vi "XY_coordinate.vi"(7 "stc_TimeInit":T4) -> (0 "str_ElapsedTime":string, 1 "str_2ndLineTime":string, 2 "str_1stLineTime":string, 3 "XY_Coordinate":picture, 4 "str_RunningTime":string, 8 "ms16EachXYHigh":i16, 9 "mu08ObjectNum":u8, 10 "mu08XOffset":u8, 11 "stc_NumOffset":cluster{"XOffset":u8, "YOffset":u8})   [LabVIEW 2011]
uses:
  <vilib>/picture/picture.llb/imagedata.ctl
panel:
  out "大小":i32
  out "image data":T1 caption="图像数据"
  out "PicJpgPath":path
  out "mbfUpdate":bool
  in  "ClearRedBlueLine":bool
  out "stc_absLine":cluster{"absTop":u8, "absBotton":u16}
  out "stc_BlueLineBK":T2
  out "stc_RedLineBK":T2
  out "stc_XYOriginOffset":T3
  out "stc_BlueLine":T2
  out "stc_RedLine":T2
  out "strInputInit":string
  out "Pic_Right":u32
  out "Pic_Left":i32
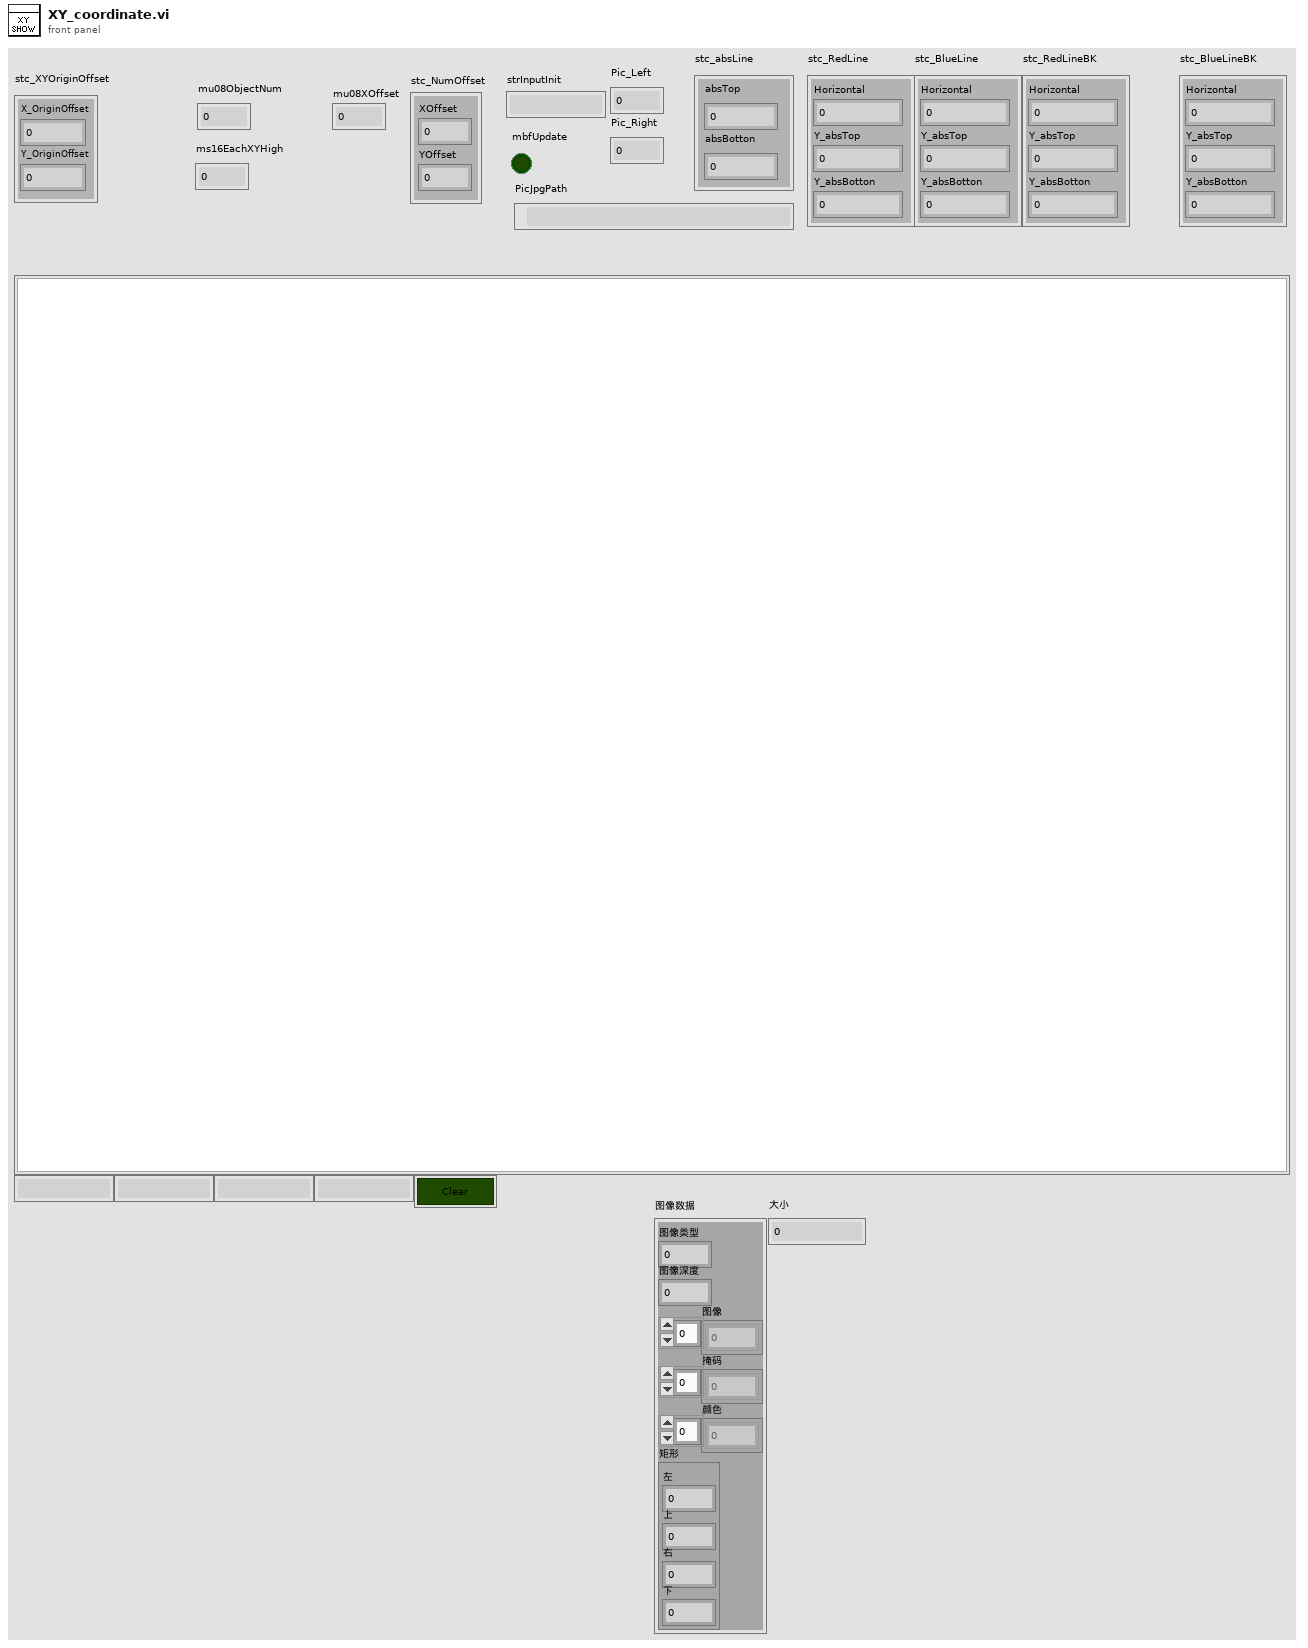
[diagram p1: front panel]
types:
  T1 = typedef "imagedata.ctl" = cluster{"image type":i32, "image depth":i32, "image":u8[], "mask":u8[], "colors":u32[], "Rectangle":cluster{"left":i16, "top":i16, "right":i16, "bottom":i16}}
  T2 = cluster{"Horizontal":u32, "Y_absTop":u8, "Y_absBotton":u16}
  T3 = cluster{"X_OriginOffset":u8, "Y_OriginOffset":dbl}
  T4 = cluster{"str_1stLineTime":string, "str_2ndLineTime":string, "str_ElapsedTime":string, "str_RunningTime":string}
  T5 = cluster{"Width":u16, "Style":enum32{"Solid", "Dash", "Dot", "DashDot", "DashDotDot"}}
  T6 = typedef "LVBoundsTypeDef.ctl" = cluster{"Width":u32, "Height":u32}
  T7 = typedef "LVPoint32TypeDef.ctl" = cluster{"Horizontal":i32, "Vertical":i32}
  T8 = cluster{"Shift":bool, "Ctrl":bool, "Alt":bool, "Cmd":bool, "Opt":bool}
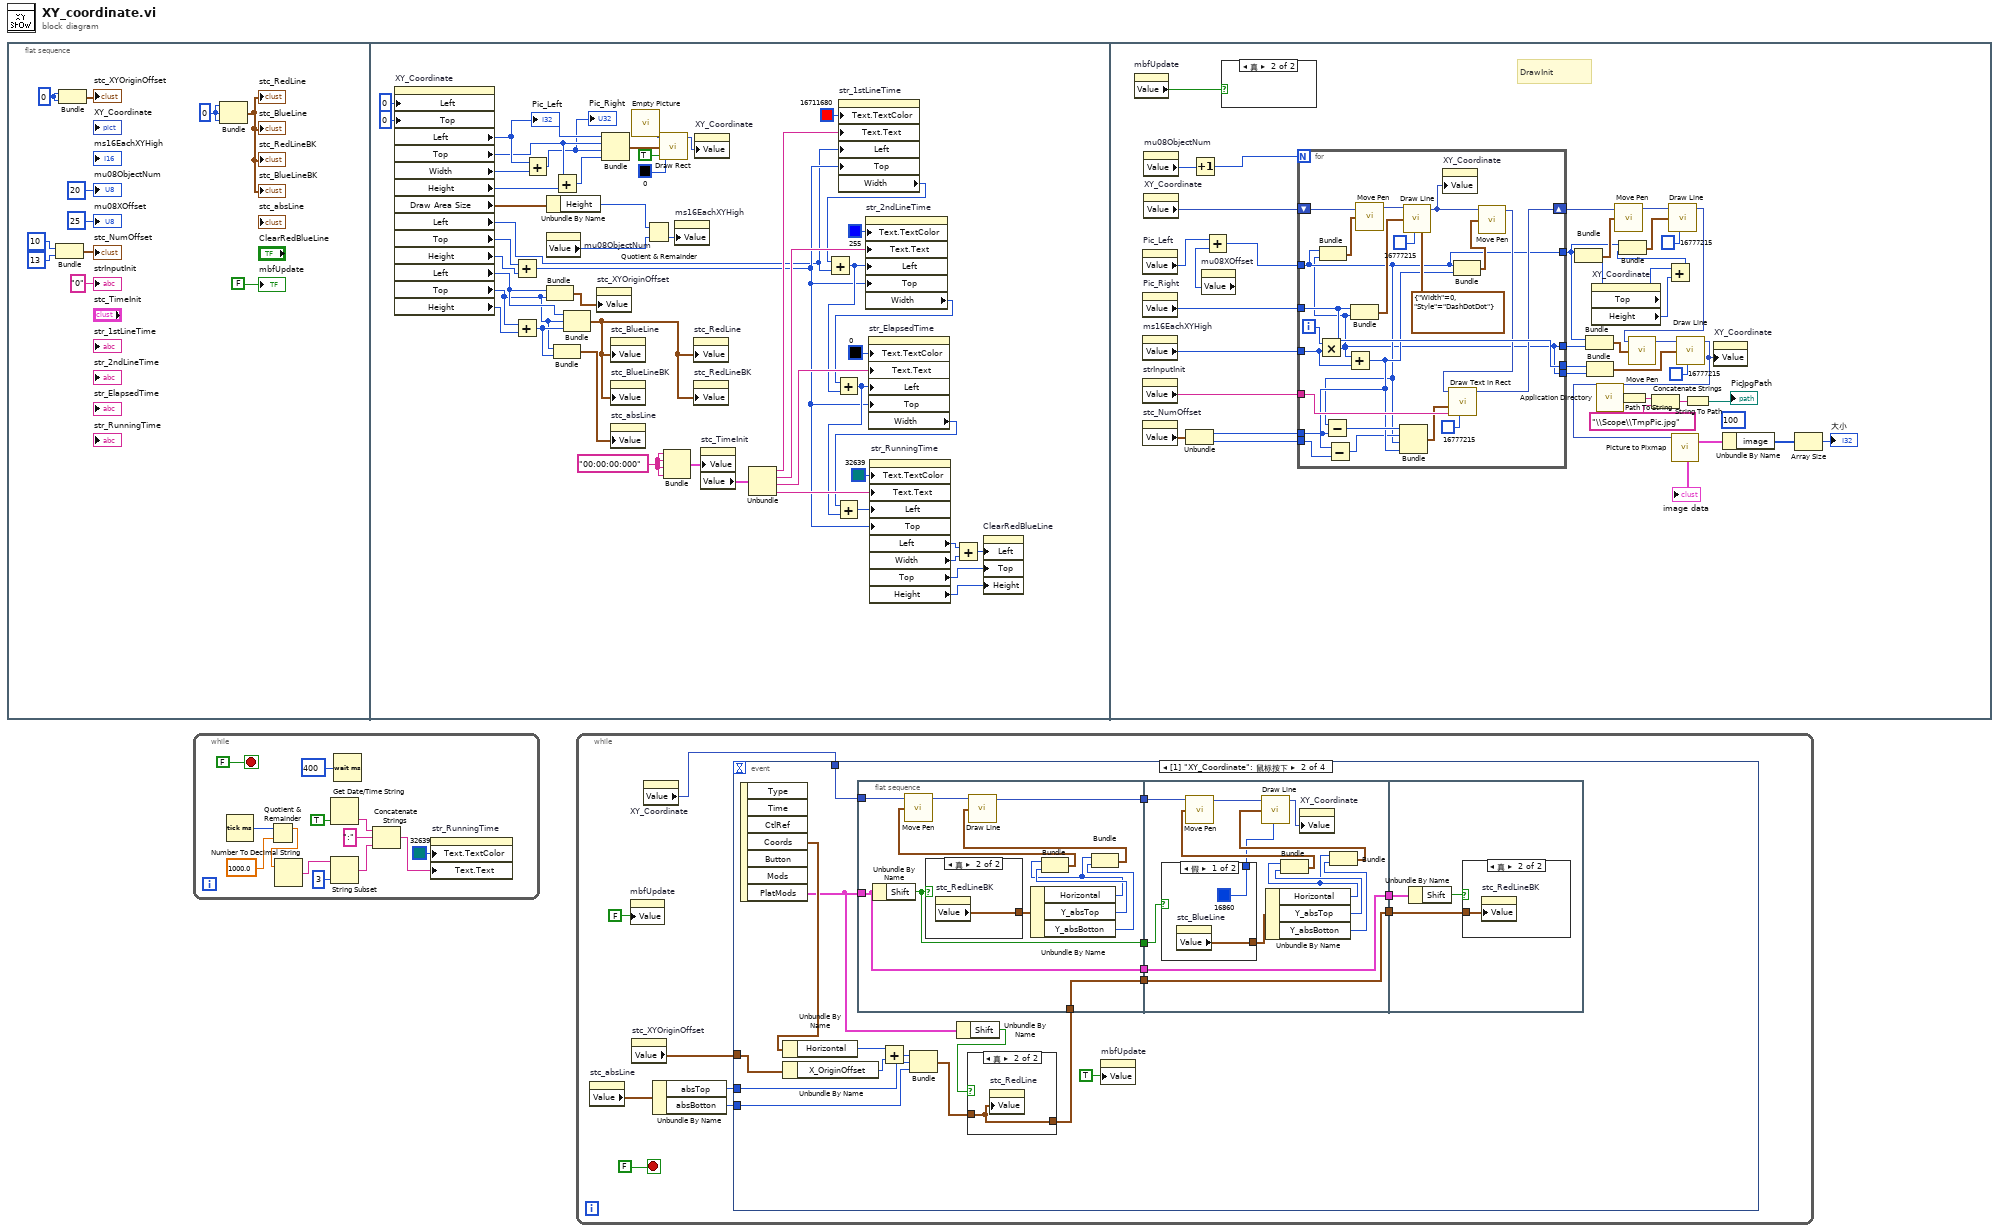
[diagram p0: block diagram]
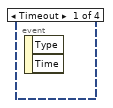
[diagram p2: hidden frame]
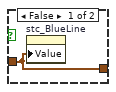
[diagram p3: hidden frame]
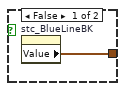
[diagram p4: hidden frame]
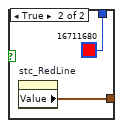
[diagram p5: hidden frame]
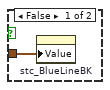
[diagram p6: hidden frame]
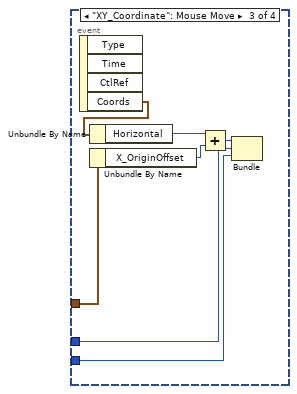
[diagram p7: hidden frame]
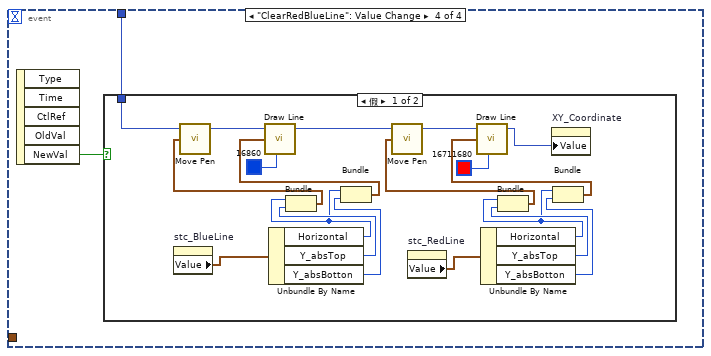
[diagram p8: hidden frame]
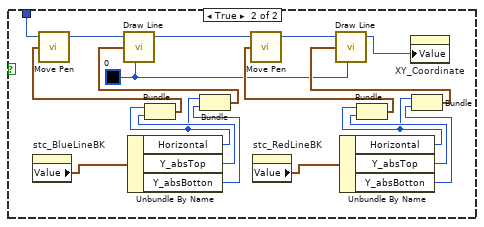
[diagram p9: hidden frame]
diagram:
  n1 = flat-sequence {
    frame #0 {
      w5 = 0
      w3 = 0
      n2 = Bundle(10, 13) -> (→"stc_NumOffset":cluster{i32, i32})  [unwired: 1 in]
      n3 = Bundle(w5, w5) -> (→"stc_XYOriginOffset":cluster{i32, i32})  [unwired: 1 in]
      n4 = Bundle(w3, w3, w3) -> (→"stc_RedLine" →"stc_BlueLine" →"stc_RedLineBK" →"stc_BlueLineBK":cluster{i32, i32, i32})  [unwired: 1 in]
      "mu08ObjectNum" <- u8 20 ("mu08ObjectNum")
      "mu08XOffset" <- u8 25 ("mu08XBuf")
      "strInputInit" <- "0" ("strInputInit")
      "mbfUpdate" <- FALSE
    }
    frame #1 {
      w43 = "00:00:00:000"
      n5 = property on="XY_Coordinate" class="Pict"("Left"=0 ("位置:居左"), "Top"=0 ("位置:置顶")) -> ("Left"=w58:i32, "Top"=w55:i32, "Width"=w57:u32, "Height"=w56:u32, "Draw Area Size"=w49:T6, "Left"=w19:i32, "Top"=w44:i32, "Height"=w18:u32, "Left"=w24:i32, "Top"=w20:i32, "Height"=w17:u32)  [unwired: 2 in, 2 out]
      "Pic_Left" <- w58
      n6 = Add(x=w44, y=w18) -> (x+y=w26:u32)
      n7 = Add(x=w20, y=w17) -> (x+y=w22:u32)
      n8 = Add(x=w58, y=w57) -> (x+y=w45:u32)
      "Pic_Right" <- w45
      n9 = Unbundle By Name(w49) -> ("Height"=w48:u32)
      n10 = property on="mu08ObjectNum" class="DigNum (严格)"() -> ("Value"=w47:u8)  [unwired: 2 in, 2 out]
      n11 = Bundle("Left"=w24, "Top"=w20) -> (w25:cluster{"Left":i32, "Top":i32})  [unwired: 1 in]
      n12 = Add(x=w55, y=w56) -> (x+y=w54:u32)
      n13 = Bundle("Top"=w20, w22) -> (w21:cluster{"Top":i32, u32})  [unwired: 1 in]
      n14 = Bundle("Left"=w24, "Top"=w20, w22) -> (w23:cluster{"Left":i32, "Top":i32, u32})  [unwired: 1 in]
      n15 = property on="stc_XYOriginOffset" class="Clust (严格)"("Value"=w25) -> ()  [unwired: 2 in, 2 out]
      n16 = Bundle("Left"=w58, "Top"=w55, w45, w54) -> (w53:cluster{"Left":i32, "Top":i32, u32, u32})  [unwired: 1 in]
      n17 = property on="stc_BlueLine" class="Clust (严格)"("Value"=w23) -> ()  [unwired: 2 in, 2 out]
      n18 = property on="stc_BlueLineBK" class="Clust (严格)"("Value"=w23) -> ()  [unwired: 2 in, 2 out]
      n19 = property on="stc_absLine" class="Clust (严格)"("Value"=w21) -> ()  [unwired: 2 in, 2 out]
      n20 = call "Empty Picture"() -> ("empty picture"=w59:picture)
      n21 = Quotient & Remainder(x=w48, y=w47) -> (floor(x/y)=w46:u32)  [unwired: 1 out]
      n22 = call <vilib>:"Draw Rect.vi"("picture"=w59, "rect"=w53, "fill?(F)"=TRUE, "color(black)"=u32 0) -> ("new picture"=w50:picture)  [unwired: 5 in]
      n23 = Bundle(w43, w43, w43, w43) -> (w42:cluster{string, string, string, string})  [unwired: 1 in]
      n24 = property on="ms16EachXYHigh" class="DigNum (严格)"("Value"=w46) -> ()  [unwired: 2 in, 2 out]
      n25 = property on="stc_RedLine" class="Clust (严格)"("Value"=w23) -> ()  [unwired: 2 in, 2 out]
      n26 = property on="stc_RedLineBK" class="Clust (严格)"("Value"=w23) -> ()  [unwired: 2 in, 2 out]
      n27 = property on="XY_Coordinate" class="Pict"("Value"=w50) -> ()  [unwired: 2 in, 2 out]
      n28 = property on="stc_TimeInit" class="Clust (严格)"("Value"=w42) -> ("Value"=w41:T4)  [unwired: 2 in, 2 out]
      n29 = Unbundle(w41) -> ("str_1stLineTime"=w36:string, "str_2ndLineTime"=w35:string, "str_ElapsedTime"=w34:string, "str_RunningTime"=w33:string)
      n30 = property on="str_1stLineTime" class="Str"("Text.TextColor"=u32 16711680, "Text.Text"=w36, "Left"=w19, "Top"=w26) -> ("Width"=w32:u32)  [unwired: 2 in, 2 out]
      n31 = Add(x=w32, y=w19) -> (x+y=w30:u32)
      n32 = property on="str_2ndLineTime" class="Str"("Text.TextColor"=u32 255, "Text.Text"=w35, "Left"=w30, "Top"=w26) -> ("Width"=w31:u32)  [unwired: 2 in, 2 out]
      n33 = Add(x=w31, y=w30) -> (x+y=w27:u32)
      n34 = property on="str_ElapsedTime" class="Str"("Text.TextColor"=u32 0, "Text.Text"=w34, "Left"=w27, "Top"=w26) -> ("Width"=w28:u32)  [unwired: 2 in, 2 out]
      n35 = Add(x=w28, y=w27) -> (x+y=w29:u32)
      n36 = property on="str_RunningTime" class="Str"("Text.TextColor"=u32 32639, "Text.Text"=w33, "Left"=w29, "Top"=w26) -> ("Left"=w15:i32, "Width"=w16:u32, "Top"=w13:i32, "Height"=w12:u32)  [unwired: 2 in, 2 out]
      n37 = Add(x=w15, y=w16) -> (x+y=w14:u32)
      n38 = property on="ClearRedBlueLine" class="Bool"("Left"=w14, "Top"=w13, "Height"=w12) -> ()  [unwired: 2 in, 2 out]
    }
    frame #2 {
      (unwired) 100 ("quality (80)")
      # "DrawInit"
      n39 = property on="mbfUpdate" class="Bool (严格)"() -> ("Value"=w100:bool)  [unwired: 2 in, 2 out]
      n40 = property on="Pic_Left" class="DigNum (严格)"() -> ("Value"=w96:i32)  [unwired: 2 in, 2 out]
      n41 = property on="Pic_Right" class="DigNum (严格)"() -> ("Value"=w99:u32)  [unwired: 2 in, 2 out]
      n42 = property on="ms16EachXYHigh" class="DigNum (严格)"() -> ("Value"=w98:i16)  [unwired: 2 in, 2 out]
      n43 = property on="strInputInit" class="Str"() -> ("Value"=w78:string)  [unwired: 2 in, 2 out]
      n44 = property on="stc_NumOffset" class="Clust (严格)"() -> ("Value"=w75:cluster{"XOffset":u8, "YOffset":u8})  [unwired: 2 in, 2 out]
      n45 = property on="mu08ObjectNum" class="DigNum (严格)"() -> ("Value"=w77:u8)  [unwired: 2 in, 2 out]
      n46 = property on="XY_Coordinate" class="Pict"() -> ("Value"=w71:picture)  [unwired: 2 in, 2 out]
      n47 = Unbundle(w75) -> ("XOffset"=w74:u8, "YOffset"=w73:u8)
      n48 = Increment(x=w77) -> (x+1=w76:u8)
      n49 = property on="mu08XOffset" class="DigNum (严格)"() -> ("Value"=w97:u8)  [unwired: 2 in, 2 out]
      n50 = Add(x=w96, y=w97) -> (x+y=w95:i32)
      n51 = case shown="真" w100 {
        frame False {
        }
        frame True {
        }
      }
      n52 = for {
        N: w76 -> [_]
        shift-right: [w116] -> w93
        shift-left: w71 -> [w103]
        tunnel: w95 -> [w105]
        tunnel: w99 -> [w117]
        tunnel: w98 -> [w119]
        tunnel: [w105] -> w85
        tunnel: [w104] -> w83
        tunnel: [w117] -> w82
        tunnel: [w104] -> w81
        tunnel: w78 -> [w114]
        tunnel: [w112] -> _
        tunnel: w74 -> [w112]
        tunnel: w73 -> [w110]
        i -> [w123]
        n53 = Multiply(x=w123, y=w119) -> (x*y=w104:i32)
        n54 = Bundle(w105, w104) -> (w101:cluster{i32, i32})  [unwired: 1 in]
        n55 = Subtract(x=w105, y=w112) -> (x-y=w111:i32)
        n56 = Add(x=w104, y=w119) -> (x+y=w109:i32)
        n57 = Subtract(x=w109, y=w110) -> (x-y=w108:i32)
        n58 = Bundle("Value"=w117, w104) -> (w118:cluster{"Value":u32, i32})  [unwired: 1 in]
        n59 = call <vilib>:"Move Pen.vi"("new position"=w101, "picture"=w103) -> ("new picture"=w102:picture)  [unwired: 3 in]
        n60 = Bundle(w111, w108, w105, w109) -> (w107:cluster{i32, i32, i32, i32})  [unwired: 1 in]
        n61 = call <vilib>:"Draw Line.vi"("picture"=w102, "end point"=w118, "color(black)"=u32 16777215, "pen"=T5 {"Width"=0, "Style"=enum."DashDotDot"}) -> ("new picture"=w121:picture)  [unwired: 5 in]
        n62 = property on="XY_Coordinate" class="Pict"("Value"=w121) -> ()  [unwired: 2 in, 2 out]
        n63 = Bundle(w105, w109) -> (w106:cluster{i32, i32})  [unwired: 1 in]
        n64 = call <vilib>:"Move Pen.vi"("new position"=w106, "picture"=w121) -> ("new picture"=w113:picture)  [unwired: 3 in]
        n65 = call <vilib>:"Draw Text in Rect.vi"("text color(black)"=u32 16777215 ("color(black)"), "text"=w114, "rect"=w107, "picture"=w113) -> ("new picture"=w116:picture)  [unwired: 7 in]
      }
      n66 = Bundle(w85, w83) -> (w80:cluster{i32, i32})  [unwired: 1 in]
      n67 = Bundle("Value"=w82, w81) -> (w79:cluster{"Value":u32, i32})  [unwired: 1 in]
      n68 = property on="XY_Coordinate" class="Pict"() -> ("Top"=w90:i32, "Height"=w87:u32)  [unwired: 2 in, 2 out]
      n69 = Bundle(w85, "Top"=w90) -> (w91:cluster{i32, "Top":i32})  [unwired: 1 in]
      n70 = call <vilib>:"Application Directory.vi"() -> ("Application Directory"=w69:path)
      n71 = call <vilib>:"Move Pen.vi"("new position"=w91, "picture"=w93) -> ("new picture"=w92:picture)  [unwired: 3 in]
      n72 = Path To String(path=w69) -> (string=w68:string)
      n73 = Concatenate Strings(w68, "\\Scope\\TmpPic.jpg") -> (w66:string)
      n74 = Add(x=w90, y=w87) -> (x+y=w88:u32)
      n75 = Bundle(w85, w88) -> (w89:cluster{i32, u32})  [unwired: 1 in]
      n76 = call <vilib>:"Draw Line.vi"("picture"=w92, "end point"=w89, "color(black)"=u32 16777215) -> ("new picture"=w72:picture)  [unwired: 6 in]
      n77 = call <vilib>:"Move Pen.vi"("new position"=w80, "picture"=w72) -> ("new picture"=w86:picture)  [unwired: 3 in]
      n78 = call <vilib>:"Draw Line.vi"("picture"=w86, "end point"=w79, "color(black)"=u32 16777215) -> ("new picture"=w70:picture)  [unwired: 6 in]
      n79 = call <vilib>:"Picture to Pixmap.vi"("picture"=w70) -> ("image data"=w64:T1)  [unwired: 9 in, 1 out]
      "image data" <- w64
      n80 = String To Path(string=w66) -> (path=→"PicJpgPath":path)
      n81 = property on="XY_Coordinate" class="Pict"("Value"=w70) -> ()  [unwired: 2 in, 2 out]
      n82 = Unbundle By Name(w64) -> ("image"=w63:u8[])
      n83 = Array Size(array=w63) -> (size(s)=→"大小":i32)
    }
  }
  n84 = while {
    stop <- FALSE stop-if-true
    n85 = Tick Count (ms)() -> (millisecond timer value=w125:u32)
    n86 = Quotient & Remainder(x=w125, y=1000.0) -> (x-y*floor(x/y)=w124:dbl)  [unwired: 1 out]
    n87 = Number To Decimal String(number=w124) -> (decimal integer string=w135:string)  [unwired: 1 in]
    n88 = Get Date/Time String(want seconds? (F)=TRUE ("需要秒？(F)")) -> (time string=w132:string)  [unwired: 2 in, 1 out]
    n89 = String Subset(string=w135, length (rest)=3 ("长度（剩余）")) -> (substring=w127:string)  [unwired: 1 in]
    n90 = Wait (ms)(milliseconds to wait=u32 400 ("等待时间（毫秒）")) -> ()  [unwired: 1 out]
    n91 = Concatenate Strings(w132, ":" ("字符串"), w127) -> (w130:string)
    n92 = property on="str_RunningTime" class="Str"("Text.TextColor"=u32 32639, "Text.Text"=w130) -> ()  [unwired: 2 in, 2 out]
  }
  n93 = while {
    stop <- FALSE stop-if-true
    n94 = property on="stc_absLine" class="Clust (严格)"() -> ("Value"=w141:cluster{"absTop":u8, "absBotton":u16})  [unwired: 2 in, 2 out]
    n95 = property on="mbfUpdate" class="Bool (严格)"("Value"=FALSE ("mbfUpdate")) -> ()  [unwired: 2 in, 2 out]
    n96 = property on="stc_XYOriginOffset" class="Clust (严格)"() -> ("Value"=w142:T3)  [unwired: 2 in, 2 out]
    n97 = property on="XY_Coordinate" class="Pict"() -> ("Value"=w138:picture)  [unwired: 2 in, 2 out]
    n98 = Unbundle By Name(w141) -> ("absTop"=w140:u8, "absBotton"=w139:u16)
    n99 = event shown="[1] \"XY_Coordinate\": 鼠标按下" {
      selector: _ -> [_ _ _ _]
      dyn-events: _ -> [_ _ _ _]
      timeout: _ -> [_ _ _ _]
      tunnel: w142 -> [_ w159 w207 _]
      tunnel: w140 -> [_ w158 w202 _]
      tunnel: w139 -> [_ w157 w201 _]
      tunnel: w138 -> [_ w155 _ w208]
      event Timeout {
        n100 = event-data() -> ()  [unwired: 1 in, 2 out]
      }
      event "XY_Coordinate": Mouse Down {
        n101 = event-data() -> ("Coords"=w160:T7, "PlatMods"=w152:T8)  [unwired: 1 in, 5 out]
        n102 = Unbundle By Name(w160) -> ("Horizontal"=w156:i32)
        n103 = Unbundle By Name(w159) -> ("X_OriginOffset"=w162:u8)
        n104 = flat-sequence {
          tunnel: w155 -> [w176]
          tunnel: w152 -> [w166]
          tunnel: [w168] -> w154
          tunnel: [w167] -> w153
          tunnel: [w166] -> w149
          tunnel: [w165] -> w146
          tunnel: w145 -> [w165]
          tunnel: w154 -> [w191]
          tunnel: w153 -> [w190]
          tunnel: w149 -> [w180]
          tunnel: [w180] -> w148
          tunnel: [w179] -> w147
          tunnel: w146 -> [w179]
          tunnel: w148 -> [w198]
          tunnel: w147 -> [w196]
          frame #0 {
            n105 = Unbundle By Name(w166) -> ("Shift"=w167:bool)
            n106 = case shown="真" w167 {
              tunnel: [w177 w178] -> w175
              frame False {
                n107 = property on="stc_BlueLineBK" class="Clust (严格)"() -> ("Value"=w177:T2)  [unwired: 2 in, 2 out]
              }
              frame True {
                n108 = property on="stc_RedLineBK" class="Clust (严格)"() -> ("Value"=w178:T2)  [unwired: 2 in, 2 out]
              }
            }
            n109 = Unbundle By Name(w175) -> ("Horizontal"=w170:u32, "Y_absTop"=w174:u8, "Y_absBotton"=w171:u16)
            n110 = Bundle("Horizontal"=w170, "Y_absTop"=w174) -> (w173:cluster{"Horizontal":u32, "Y_absTop":u8})  [unwired: 1 in]
            n111 = call <vilib>:"Move Pen.vi"("new position"=w173, "picture"=w176) -> ("new picture"=w172:picture)  [unwired: 3 in]
            n112 = Bundle("Horizontal"=w170, "Y_absBotton"=w171) -> (w169:cluster{"Horizontal":u32, "Y_absBotton":u16})  [unwired: 1 in]
            n113 = call <vilib>:"Draw Line.vi"("picture"=w172, "end point"=w169) -> ("new picture"=w168:picture)  [unwired: 7 in]
          }
          frame #1 {
            n114 = case shown="假" w190 {
              tunnel: [w193 w195] -> w189
              tunnel: [u32 16860 u32 16711680 ("color(black)")] -> w181
              frame False {
                n115 = property on="stc_BlueLine" class="Clust (严格)"() -> ("Value"=w193:T2)  [unwired: 2 in, 2 out]
              }
              frame True {
                n116 = property on="stc_RedLine" class="Clust (严格)"() -> ("Value"=w195:T2)  [unwired: 2 in, 2 out]
              }
            }
            n117 = Unbundle By Name(w189) -> ("Horizontal"=w186:u32, "Y_absTop"=w187:u8, "Y_absBotton"=w185:u16)
            n118 = Bundle("Horizontal"=w186, "Y_absTop"=w187) -> (w188:cluster{"Horizontal":u32, "Y_absTop":u8})  [unwired: 1 in]
            n119 = call <vilib>:"Move Pen.vi"("new position"=w188, "picture"=w191) -> ("new picture"=w183:picture)  [unwired: 3 in]
            n120 = Bundle("Horizontal"=w186, "Y_absBotton"=w185) -> (w184:cluster{"Horizontal":u32, "Y_absBotton":u16})  [unwired: 1 in]
            n121 = call <vilib>:"Draw Line.vi"("picture"=w183, "end point"=w184, "color(black)"=w181) -> ("new picture"=w182:picture)  [unwired: 6 in]
            n122 = property on="XY_Coordinate" class="Pict"("Value"=w182) -> ()  [unwired: 2 in, 2 out]
          }
          frame #2 {
            n123 = Unbundle By Name(w198) -> ("Shift"=w197:bool)
            n124 = case shown="真" w197 {
              tunnel: w196 -> [w199 w200]
              frame False {
                n125 = property on="stc_BlueLineBK" class="Clust (严格)"("Value"=w199) -> ()  [unwired: 2 in, 2 out]
              }
              frame True {
                n126 = property on="stc_RedLineBK" class="Clust (严格)"("Value"=w200) -> ()  [unwired: 2 in, 2 out]
              }
            }
          }
        }
        n127 = Add(x=w156, y=w162) -> (x+y=w161:i32)
        n128 = Bundle(w161, "absTop"=w158, "absBotton"=w157) -> (w150:cluster{i32, "absTop":u8, "absBotton":u16})  [unwired: 1 in]
        n129 = Unbundle By Name(w152) -> ("Shift"=w151:bool)
        n130 = case shown="真" w151 {
          tunnel: w150 -> [w163 w164]
          tunnel: [w163 w164] -> w145
          frame False {
            n131 = property on="stc_BlueLine" class="Clust (严格)"("Value"=w163) -> ()  [unwired: 2 in, 2 out]
          }
          frame True {
            n132 = property on="stc_RedLine" class="Clust (严格)"("Value"=w164) -> ()  [unwired: 2 in, 2 out]
          }
        }
        n133 = property on="mbfUpdate" class="Bool (严格)"("Value"=TRUE ("mbfUpdate")) -> ()  [unwired: 2 in, 2 out]
      }
      event "XY_Coordinate": Mouse Move {
        n134 = event-data() -> ("Coords"=w206:T7)  [unwired: 1 in, 3 out]
        n135 = Unbundle By Name(w206) -> ("Horizontal"=w204:i32)
        n136 = Unbundle By Name(w207) -> ("X_OriginOffset"=w205:u8)
        n137 = Add(x=w204, y=w205) -> (x+y=w203:i32)
        n138 = Bundle(w203, "absTop"=w202, "absBotton"=w201) -> ()  [unwired: 1 in, 1 out]
      }
      event "ClearRedBlueLine": Value Change {
        n139 = event-data() -> ("NewVal"=w209:bool)  [unwired: 1 in, 4 out]
        n140 = case shown="假" w209 {
          tunnel: w208 -> [w212 w241]
          frame False {
            n141 = property on="stc_BlueLine" class="Clust (严格)"() -> ("Value"=w222:T2)  [unwired: 2 in, 2 out]
            n142 = Unbundle By Name(w222) -> ("Horizontal"=w226:u32, "Y_absTop"=w227:u8, "Y_absBotton"=w225:u16)
            n143 = Bundle("Horizontal"=w226, "Y_absTop"=w227) -> (w228:cluster{"Horizontal":u32, "Y_absTop":u8})  [unwired: 1 in]
            n144 = call <vilib>:"Move Pen.vi"("new position"=w228, "picture"=w212) -> ("new picture"=w223:picture)  [unwired: 3 in]
            n145 = Bundle("Horizontal"=w226, "Y_absBotton"=w225) -> (w224:cluster{"Horizontal":u32, "Y_absBotton":u16})  [unwired: 1 in]
            n146 = call <vilib>:"Draw Line.vi"("picture"=w223, "end point"=w224, "color(black)"=u32 16860) -> ("new picture"=w215:picture)  [unwired: 6 in]
            n147 = property on="stc_RedLine" class="Clust (严格)"() -> ("Value"=w216:T2)  [unwired: 2 in, 2 out]
            n148 = Unbundle By Name(w216) -> ("Horizontal"=w219:u32, "Y_absTop"=w220:u8, "Y_absBotton"=w218:u16)
            n149 = Bundle("Horizontal"=w219, "Y_absTop"=w220) -> (w221:cluster{"Horizontal":u32, "Y_absTop":u8})  [unwired: 1 in]
            n150 = call <vilib>:"Move Pen.vi"("new position"=w221, "picture"=w215) -> ("new picture"=w214:picture)  [unwired: 3 in]
            n151 = Bundle("Horizontal"=w219, "Y_absBotton"=w218) -> (w217:cluster{"Horizontal":u32, "Y_absBotton":u16})  [unwired: 1 in]
            n152 = call <vilib>:"Draw Line.vi"("picture"=w214, "end point"=w217, "color(black)"=u32 16711680) -> ("new picture"=w213:picture)  [unwired: 6 in]
            n153 = property on="XY_Coordinate" class="Pict"("Value"=w213) -> ()  [unwired: 2 in, 2 out]
          }
          frame True {
            w229 = u32 0
            n154 = property on="stc_BlueLineBK" class="Clust (严格)"() -> ("Value"=w239:T2)  [unwired: 2 in, 2 out]
            n155 = Unbundle By Name(w239) -> ("Horizontal"=w244:u32, "Y_absTop"=w245:u8, "Y_absBotton"=w243:u16)
            n156 = Bundle("Horizontal"=w244, "Y_absTop"=w245) -> (w246:cluster{"Horizontal":u32, "Y_absTop":u8})  [unwired: 1 in]
            n157 = call <vilib>:"Move Pen.vi"("new position"=w246, "picture"=w241) -> ("new picture"=w240:picture)  [unwired: 3 in]
            n158 = Bundle("Horizontal"=w244, "Y_absBotton"=w243) -> (w242:cluster{"Horizontal":u32, "Y_absBotton":u16})  [unwired: 1 in]
            n159 = call <vilib>:"Draw Line.vi"("picture"=w240, "end point"=w242, "color(black)"=w229) -> ("new picture"=w232:picture)  [unwired: 6 in]
            n160 = property on="stc_RedLineBK" class="Clust (严格)"() -> ("Value"=w233:T2)  [unwired: 2 in, 2 out]
            n161 = Unbundle By Name(w233) -> ("Horizontal"=w236:u32, "Y_absTop"=w237:u8, "Y_absBotton"=w235:u16)
            n162 = Bundle("Horizontal"=w236, "Y_absTop"=w237) -> (w238:cluster{"Horizontal":u32, "Y_absTop":u8})  [unwired: 1 in]
            n163 = call <vilib>:"Move Pen.vi"("new position"=w238, "picture"=w232) -> ("new picture"=w231:picture)  [unwired: 3 in]
            n164 = Bundle("Horizontal"=w236, "Y_absBotton"=w235) -> (w234:cluster{"Horizontal":u32, "Y_absBotton":u16})  [unwired: 1 in]
            n165 = call <vilib>:"Draw Line.vi"("picture"=w231, "end point"=w234, "color(black)"=w229) -> ("new picture"=w230:picture)  [unwired: 6 in]
            n166 = property on="XY_Coordinate" class="Pict"("Value"=w230) -> ()  [unwired: 2 in, 2 out]
          }
        }
      }
    }
  }
